vi "Thorlabs Module.vi"(7 "Actions":T3(ring)=enum."Start Acquire", 8 "error in":errorcluster, 9 "Objective":u16(ring)=1 items=["5X LKM05", "10X LKM10", "20X LKM20", "10X LSM02"], 10 "ROI Parameters":T1={"ROI (mm)"={"X (mm)"=1.0, "Y (mm)"=1.0}, "Shift (mm)"={"Xshift (mm)"=0.0, "Yshift (mm)"=0.0}}, 11 "Scan Parameters":T2={"# Scan"={"#Ascan"=400, "#Bscan"=400}, "# Rpt"={"#ARpt"=1, "#BRpt"=1}, "Aline Rate"=2, "# Extra"={"# ARpt_extra"=5, "#Brtn_extra"=60}} {"Aline Rate" items=["76 KHz", "146 KHz", "76 KHz", "28 KHz", "10 KHz"]}) -> (0 "error out":errorcluster, 3 "Data":u16[][](array[numeric]))   [LabVIEW 2017]
uses:
  Hardware/Thorlabs OCT/user.lib/SpectralRadar.llb/Scan Pattern.lvclass
  Hardware/Thorlabs OCT/user.lib/SpectralRadar.llb/Processing Flag Selection.ctl
  Hardware/Thorlabs OCT/user.lib/SpectralRadar.llb/Raw Data.lvclass
  Hardware/Thorlabs OCT/user.lib/SpectralRadar.llb/Processing.lvclass
  Hardware/Thorlabs OCT/user.lib/SpectralRadar.llb/Probe.lvclass
  Hardware/Thorlabs OCT/user.lib/SpectralRadar.llb/OCT Device.lvclass
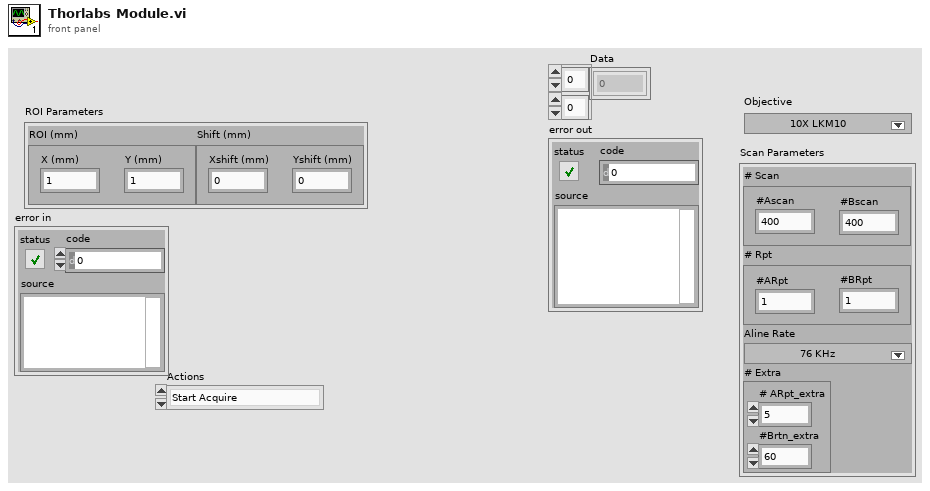
[diagram p1: front panel]
types:
  T1 = cluster{"ROI (mm)":cluster{"X (mm)":sgl, "Y (mm)":sgl}, "Shift (mm)":cluster{"Xshift (mm)":sgl, "Yshift (mm)":sgl}}
  T2 = cluster{"# Scan":cluster{"#Ascan":i32, "#Bscan":i32}, "# Rpt":cluster{"#ARpt":i32, "#BRpt":i32}, "Aline Rate":u16, "# Extra":cluster{"# ARpt_extra":i32, "#Brtn_extra":i32}}
  T3 = enum16{"Init", "Configure", "Generate Scan Pattern", "Start Acquire", "Acquire RAW", "Stop Acquire", "Uninit"}
  T4 = typedef "Processing.lvclass/Processing Flag Selection.ctl" = enum16{"Use Offset Errors", "Remove DC Spectrum", "Remove Advanced DC Spectrum", "Use Apodization", "Use Scan For Apodization", "Filter Undersampled Signals", "Use Dispersion Compensation", "Use Dechirp", "Use Extended Adjust", "Full Range Output", "Filter DC", "Autocorrelation Compensation", "DEFR", "Only Windowing", "Remove Fixed Pattern"}
  T5 = enum16{"FreeRunning", "TrigBoard_ExternalStart", "External_AScan"}
  T6 = enum16{"Asynchronous Continuous", "Asynchronous Finite", "Synchronous"}
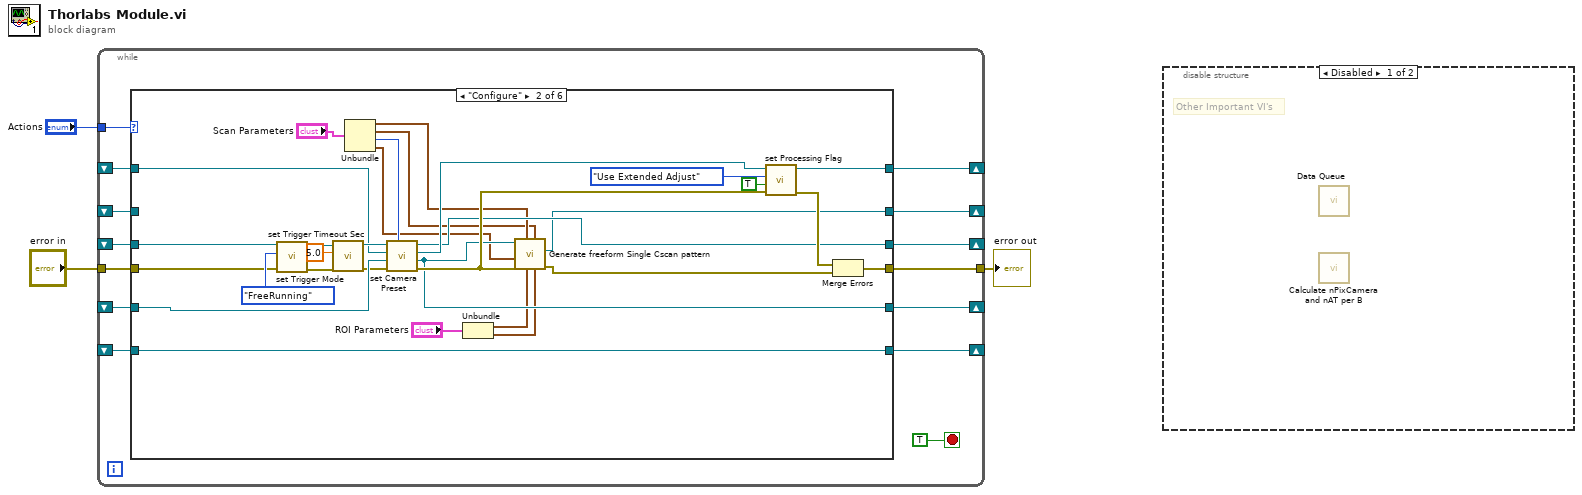
[diagram p0: block diagram]
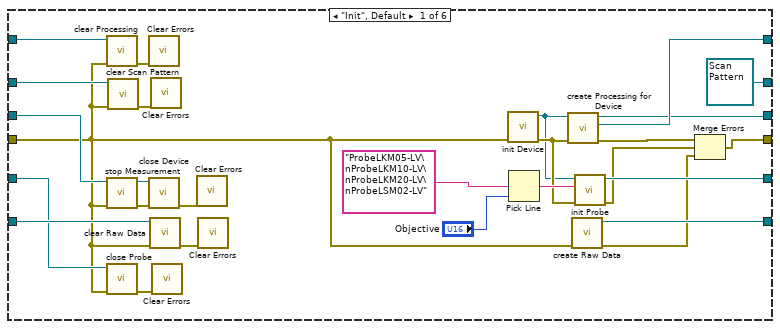
[diagram p3: hidden frame]
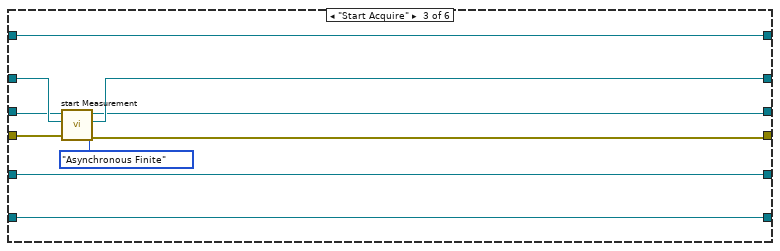
[diagram p4: hidden frame]
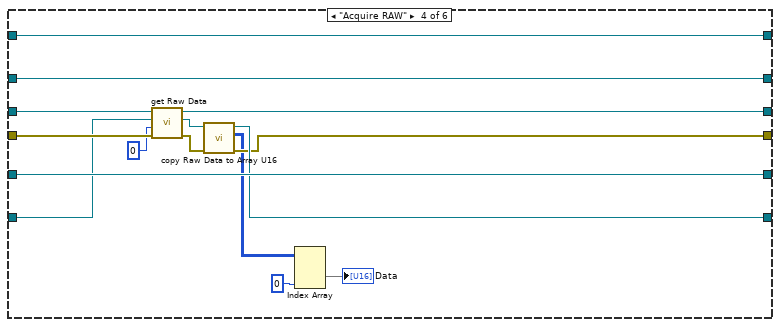
[diagram p5: hidden frame]
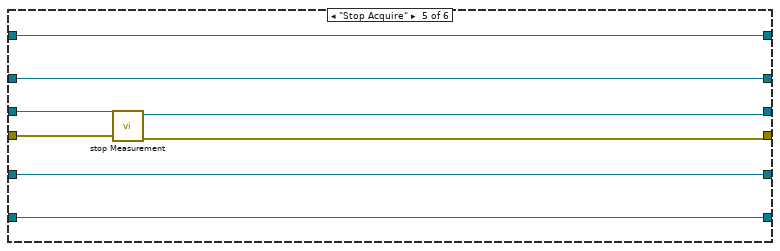
[diagram p6: hidden frame]
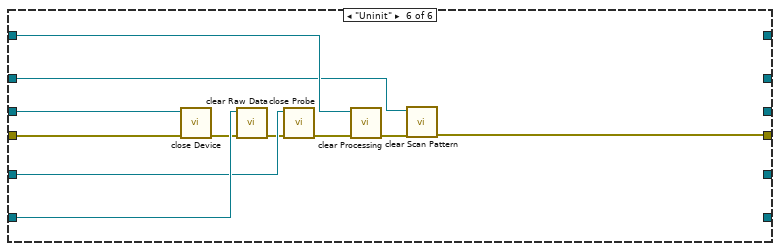
[diagram p7: hidden frame]
diagram:
  n1 = while {
    tunnel: "Actions" -> [w17]
    shift-right: [w15] -> _
    shift-left: _ -> [w11]
    shift-right: [w12] -> _
    shift-left: _ -> [w10]
    shift-right: [w9] -> _
    shift-left: _ -> [w8]
    shift-right: [w7] -> _
    shift-left: _ -> [w6]
    shift-right: [w5] -> _
    shift-left: _ -> [w4]
    tunnel: "error in" -> [w13]
    tunnel: [w14] -> w2
    stop <- TRUE stop-if-true
    n2 = case shown="\"Configure\"" w17 {
      tunnel: [w30 w58 w79 w93 w104 _] -> w15
      tunnel: [w37 w73 w83 w88 w106 w108] -> w14
      tunnel: w13 -> [w21 w46 w84 w97 w107 w115]
      tunnel: [w39 w59 w77 w98 w101 _] -> w12
      tunnel: w11 -> [w27 w45 w80 w95 w105 w116]
      tunnel: w10 -> [w24 w67 w77 w98 w101 w114]
      tunnel: [w32 w65 w78 w99 w102 _] -> w9
      tunnel: w8 -> [w22 w47 w78 w99 w102 w111]
      tunnel: [w40 w61 w76 w89 w100 _] -> w7
      tunnel: w6 -> [w25 w61 w76 w94 w100 w118]
      tunnel: [refnum<class "Scan Pattern.lvclass"> refnum ("Scan Pattern") w57 w81 w92 w103 _] -> w5
      tunnel: w4 -> [w23 _ w82 w92 w103 w109]
      frame "Init", Default {
        n3 = call "clear Processing.vi"("error in (no error)"=w21, "Processing"=w22) -> ("error out"=w20:errorcluster)  [unwired: 5 in]
        n4 = call "stop Measurement.vi"("error in (no error)"=w21, "OCTDevice"=w27) -> ("error out"=w29:errorcluster, "OCTDevice"=w28:refnum<class "OCT Device.lvclass">)  [unwired: 4 in]
        n5 = call "close Probe.vi"("error in (no error)"=w21, "GalvoControl"=w24) -> ("error out"=w19:errorcluster)  [unwired: 5 in]
        n6 = call "clear Scan Pattern.vi"("error in (no error)"=w21, "Scan Pattern in"=w23) -> ("error out"=w18:errorcluster)  [unwired: 5 in]
        n7 = call <vilib>:"Clear Errors.vi"("error in (no error)"=w20) -> ()  [unwired: 5 in, 2 out]
        n8 = call "close Device.vi"("error in (no error)"=w29, "OCTDevice"=w28) -> ("error out"=w42:errorcluster)  [unwired: 5 in]
        n9 = call "clear Raw Data.vi"("error in (no error)"=w21, "Raw Data"=w25) -> ("error out"=w41:errorcluster)  [unwired: 5 in]
        n10 = call <vilib>:"Clear Errors.vi"("error in (no error)"=w18) -> ()  [unwired: 5 in, 2 out]
        n11 = call <vilib>:"Clear Errors.vi"("error in (no error)"=w19) -> ()  [unwired: 5 in, 2 out]
        n12 = call <vilib>:"Clear Errors.vi"("error in (no error)"=w42) -> ()  [unwired: 5 in, 2 out]
        n13 = call <vilib>:"Clear Errors.vi"("error in (no error)"=w41) -> ()  [unwired: 5 in, 2 out]
        n14 = call "init Device.vi"("error in (no error)"=w21) -> ("error out"=w34:errorcluster, "OCTDevice"=w33:refnum<class "OCT Device.lvclass">)  [unwired: 5 in]
        n15 = Pick Line(multi-line string="ProbeLKM05-LV\nProbeLKM10-LV\nProbeLKM20-LV\nProbeLSM02-LV" ("string (\"\")"), line index="Objective") -> (output string=w38:string)  [unwired: 1 in]
        n16 = call "create Processing for Device.vi"("error in (no error)"=w34, "OCTDevice"=w33) -> ("error out"=w31:errorcluster, "Processing"=w32:refnum<class "Processing.lvclass">, "OCTDevice"=w30:refnum<class "OCT Device.lvclass">)  [unwired: 3 in]
        n17 = call "create Raw Data.vi"("error in (no error)"=w21) -> ("error out"=w35:errorcluster, "Raw Data"=w40:refnum<class "Raw Data.lvclass">)  [unwired: 5 in]
        n18 = call "init Probe.vi"("error in (no error)"=w34, "Probe"=w38, "OCT Device"=w33) -> ("error out"=w36:errorcluster, "GalvoControl"=w39:refnum<class "Probe.lvclass">)  [unwired: 3 in]
        n19 = Merge Errors(w31, w36, w35) -> (w37:errorcluster)
      }
      frame "Configure" {
        n20 = call "set Trigger Mode.vi"("error in (no error)"=w46, "Trigger Type"=T5."FreeRunning", "OCTDevice in"=w45) -> ("error out"=w72:errorcluster, "OCTDevice out"=w74:refnum<class "OCT Device.lvclass">)  [unwired: 3 in]
        n21 = call "set Trigger Timeout Sec.vi"("error in (no error)"=w72, "Trigger Timeout"=5.0, "OCTDevice in"=w74) -> ("error out"=w64:errorcluster, "OCTDevice out"=w63:refnum<class "OCT Device.lvclass">)  [unwired: 3 in]
        n22 = Unbundle("Scan Parameters") -> ("# Scan"=w52:cluster{"#Ascan":i32, "#Bscan":i32}, "# Rpt"=w51:cluster{"#ARpt":i32, "#BRpt":i32}, "Aline Rate"=w53:u16, "# Extra"=w48:cluster{"# ARpt_extra":i32, "#Brtn_extra":i32})
        n23 = call "set Camera Preset.vi"("Numeric"=w53, "error in (no error)"=w64, "Probe"=w67, "Processing"=w47, "OCTDevice"=w63) -> ("error out"=w60:errorcluster, "Probe 2"=w59:refnum<class "Probe.lvclass">, "Processing"=w66:refnum<class "Processing.lvclass">, "OCTDevice out"=w58:refnum<class "OCT Device.lvclass">)  [unwired: 1 in]
        n24 = Unbundle("ROI Parameters") -> ("ROI (mm)"=w50:cluster{"X (mm)":sgl, "Y (mm)":sgl}, "Shift (mm)"=w49:cluster{"Xshift (mm)":sgl, "Yshift (mm)":sgl})
        n25 = call "Generate freeform Single Cscan pattern.vi"("Shift (mm)"=w49, "# Rpt"=w51, "ROI (mm)"=w50, "# Scan"=w52, "error in (no error)"=w60, "# Extra"=w48, "Probe"=w59) -> ("error out"=w56:errorcluster, "Scan Pattern"=w57:refnum<class "Scan Pattern.lvclass">)  [unwired: 1 in, 2 out]
        n26 = call "set Processing Flag.vi"("error in (no error)"=w60, "Flag"=TRUE, "Processing Flag Selection"=Processing_Flag_Selection."Use Extended Adjust", "Processing"=w66) -> ("error out"=w62:errorcluster, "Processing"=w65:refnum<class "Processing.lvclass">)  [unwired: 2 in]
        n27 = Merge Errors(w62, w56) -> (w73:errorcluster)
      }
      frame "Start Acquire" {
        n28 = call "start Measurement.vi"("error in (no error)"=w84, "Acquisition Type"=T6."Asynchronous Finite", "Scan Pattern"=w82, "OCTDevice"=w80) -> ("error out"=w83:errorcluster, "Scan Pattern"=w81:refnum<class "Scan Pattern.lvclass">, "OCTDevice"=w79:refnum<class "OCT Device.lvclass">)  [unwired: 1 in]
      }
      frame "Acquire RAW" {
        n29 = call "get Raw Data.vi"("error in (no error)"=w97, "Camera Index"=0, "RawData in"=w94, "OCTDevice in"=w95) -> ("error out"=w91:errorcluster, "RawData out"=w90:refnum<class "Raw Data.lvclass">, "OCTDevice out"=w93:refnum<class "OCT Device.lvclass">)  [unwired: 1 in]
        n30 = call "copy Raw Data to Array U16.vi"("error in (no error)"=w91, "Data in"=w90) -> ("error out"=w88:errorcluster, "Data Content"=w86:u16[][][], "Data out"=w89:refnum<class "Raw Data.lvclass">)  [unwired: 3 in]
        n31 = Index Array(array=w86, index (dim 2)=0 ("index (page)")) -> (element=→"Data":u16[][])  [unwired: 2 in]
      }
      frame "Stop Acquire" {
        n32 = call "stop Measurement.vi"("error in (no error)"=w107, "OCTDevice"=w105) -> ("error out"=w106:errorcluster, "OCTDevice"=w104:refnum<class "OCT Device.lvclass">)  [unwired: 4 in]
      }
      frame "Uninit" {
        n33 = call "close Device.vi"("error in (no error)"=w115, "OCTDevice"=w116) -> ("error out"=w117:errorcluster)  [unwired: 5 in]
        n34 = call "clear Raw Data.vi"("error in (no error)"=w117, "Raw Data"=w118) -> ("error out"=w113:errorcluster)  [unwired: 5 in]
        n35 = call "close Probe.vi"("error in (no error)"=w113, "GalvoControl"=w114) -> ("error out"=w112:errorcluster)  [unwired: 5 in]
        n36 = call "clear Processing.vi"("error in (no error)"=w112, "Processing"=w111) -> ("error out"=w110:errorcluster)  [unwired: 5 in]
        n37 = call "clear Scan Pattern.vi"("error in (no error)"=w110, "Scan Pattern in"=w109) -> ("error out"=w108:errorcluster)  [unwired: 5 in]
      }
    }
  }
  "error out" <- w2
  n38 = disable-structure shown="Disabled" {
    frame Disabled {
      # "Other Important VI's"
      n39 = call "Data Queue.vi"() -> ()  [unwired: 10 in, 2 out]
      n40 = call "Calculate nPixCamera and nAT per B.vi"() -> ()  [unwired: 9 in, 3 out]
    }
    frame Enabled {
    }
  }
